vi "Write Wheel Run State.vi"(8 "error in (no error)":errorcluster, 9 "Run":bool=TRUE, 10 "Wheel":i32, 11 "Filter Wheel in":refnum<class "Filter Wheel.lvclass">) -> (0 "error out":errorcluster, 3 "Filter Wheel out":refnum<class "Filter Wheel.lvclass">)   [LabVIEW 2024, in "Filter Wheel.lvclass"]
uses:
  Filter Wheel.lvclass
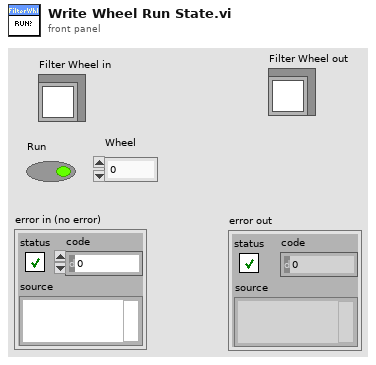
[diagram p1: front panel]
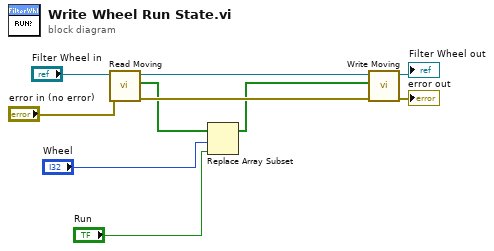
[diagram p0: block diagram]
diagram:
  n1 = call-dynamic "Read Moving.vi"("error in (no error)"="error in (no error)", "Filter Wheel in"="Filter Wheel in") -> ("error out"=w9:errorcluster, "Moving"=w5:bool[], "Filter Wheel out"=w10:refnum<class "Filter Wheel.lvclass">)  [unwired: 7 in]
  n2 = Replace Array Subset(array=w5, new element="Run", index="Wheel") -> (w2:bool[])
  n3 = call-dynamic "Write Moving.vi"("error in (no error)"=w9, "Moving"=w2, "Filter Wheel in"=w10) -> ("error out"=→"error out":errorcluster, "Filter Wheel out"=→"Filter Wheel out":refnum<class "Filter Wheel.lvclass">)  [unwired: 7 in]
